vi "dvp Vi Set Roi.vi"(6 "H":i32, 7 "W":i32, 9 "Y":i32, 10 "X":i32, 11 "handle":u32) -> (3 "function return":u32(ring))   [LabVIEW 2018, in "LabViewDVPCamera.lvlib"]
doc: "LabviewDvp2Api dvpStatus dvpViSetRoi(\n dvpHandle handle, \n dvpInt32 X,\n dvpInt32 Y,\n dvpInt32 W,\n dvpInt32 H);"
uses:
  LabViewDVPCamera.lvlib
  LabViewDVPCamera/LabViewDVPCamera.dll
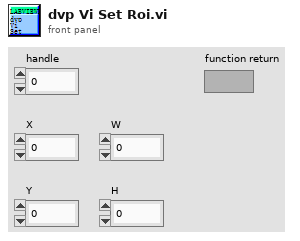
[diagram p1: front panel]
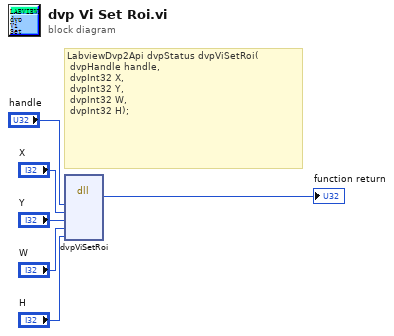
[diagram p0: block diagram]
diagram:
  # "LabviewDvp2Api dvpStatus dvpViSetRoi(\n\tdvpHandle handle, \n\tdvpInt32 X,\n\tdvpInt32 Y,\n\tdvpInt32 W,\n\tdvpInt32 H);"
  n1 = dll-call lib="C:/Program Files (x86)/DVP2 Labview cn 64/Sample/LabViewDVPCamera/LabViewDVPCamera.*" fn="dvpViSetRoi"("handle"="handle", "X"="X", "Y"="Y", "W"="W", "H"="H") -> (→"function return":u32)  [unwired: 8 in, 2 out]
